vi "Dev List - Apply New.vi"(8 "error in (no error)":errorcluster, 9 "Dev Data Lookup Table in":variant, 10 "DataGridView in":refnum<class "DataGridView.lvclass">, 11 "Controller UI in":refnum<class "Controller UI.lvclass">) -> (0 "error out":errorcluster, 1 "Dev Data Lookup Table in out":variant, 2 "DataGridView out":refnum<class "DataGridView.lvclass">)   [LabVIEW 2016, in "Controller UI.lvlib" / "Controller UI.lvclass"]
uses:
  <userlib>/Common Components/Controller UI/Controller UI.lvclass
  C:/Program Files (x86)/National Instruments/LabVIEW 2016/vi.lib/ActorFramework/Actor/Actor.lvclass
  <userlib>/LabVIEWdotNetDataGrid/source/DataGridView/DataGridView.lvclass
  <vilib>/ActorFramework/Actor/Actor.lvclass/Actor.ctl
  <vilib>/ActorFramework/Message Enqueuer/Message Enqueuer.lvclass/Message Enqueuer.ctl
  <userlib>/Common Components/Hardware/DevInfo/DevInfo.lvclass
  <userlib>/Common Components/Controller UI/Dev Variant Data.ctl
  <userlib>/Common Components/Hardware/DevInfo/DevInfo.lvclass/DevInfo.ctl
  <userlib>/Common Components/Controller/Messages/Update a Dev Requested by UI Msg/Update a Dev Requested by UI Msg.lvclass/Update a Dev Requested by UI Msg.ctl
  <userlib>/Common Components/Hardware/DevInfo/Read GUID.vi
  <vilib>/ActorFramework/Message Enqueuer/Enqueue.vi
  <userlib>/Common Components/Controller Messages/Remove All Devices Msg/Remove All Devices Msg.lvclass
  C:/Program Files (x86)/National Instruments/LabVIEW 2016/vi.lib/ActorFramework/Message/Message.lvclass
  <userlib>/Common Components/Controller/Messages/Update a Dev Requested by UI Msg/Update a Dev Requested by UI Msg.lvclass
  <vilib>/ActorFramework/Message Priority Queue/Priority Enqueue.vi
  <userlib>/LabVIEWdotNetDataGrid/source/DataGridView/Get DataArray (String).vi
  <vilib>/ActorFramework/Actor/Actor.lvclass
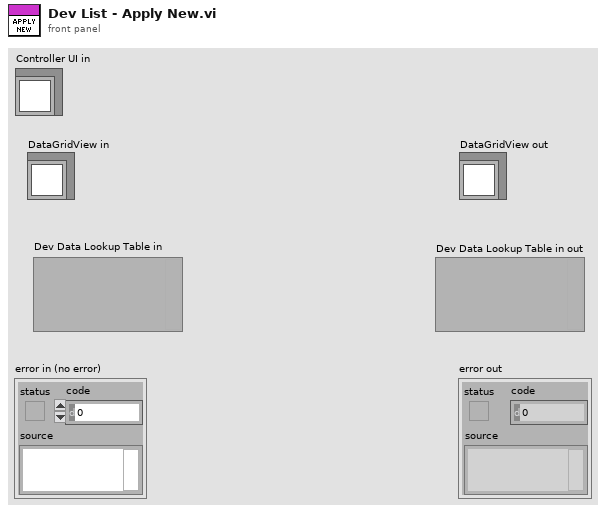
[diagram p1: front panel]
types:
  T1 = typedef "Controller UI.lvlib/Controller UI.lvclass/Dev Variant Data.ctl" = cluster{"Row Index":i32, "DevInfo Obj":refnum<class "DevInfo.lvclass">}
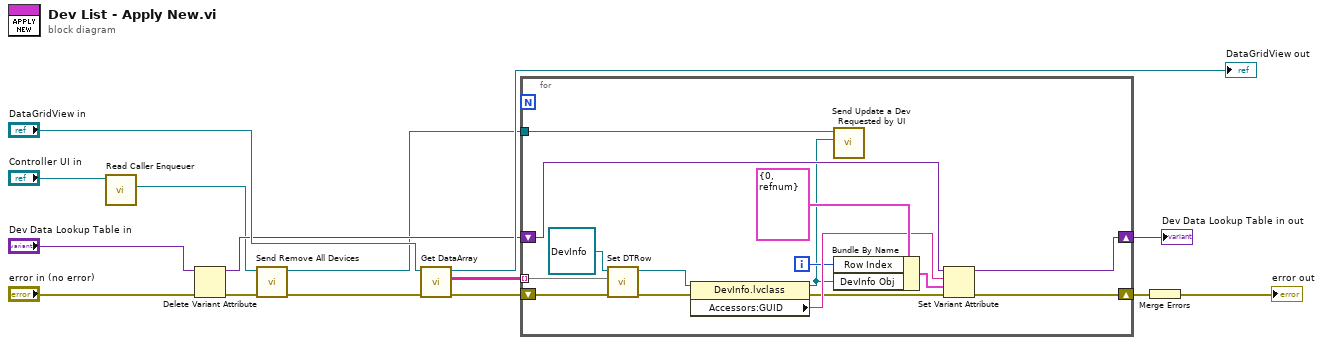
[diagram p0: block diagram]
diagram:
  n1 = call <vilib>:"Read Caller Enqueuer.vi"("Actor"="Controller UI in") -> ("Caller Enqueuer"=w2:refnum<class "Message Enqueuer.lvclass">)  [unwired: 10 in]
  n2 = Delete Variant Attribute(4:"error in (no error)", 7:"Dev Data Lookup Table in") -> (0:w6:errorcluster, 3:w9:variant)  [unwired: 1 in, 1 out]
  n3 = call <userlib>:"Send Remove All Devices.vi"("error in (no error)"=w6, "Message Enqueuer"=w2) -> ("error out"=w3:errorcluster, "Message Enqueuer out"=w1:refnum<class "Message Enqueuer.lvclass">)  [unwired: 8 in]
  n4 = call-poly <userlib>:"Get DataArray.vi"("error in (no error)"=w3, "DataGridView in"="DataGridView in") -> ("error out"=w5:errorcluster, "Array"=w14:string[][], "DataGridView out"=→"DataGridView out":refnum<class "DataGridView.lvclass">)  [unwired: 7 in]
  n5 = for {
    tunnel: w14 -> [w29] mode=indexing
    shift-right: [w19] -> w4
    shift-left: w5 -> [w27]
    shift-right: [w22] -> w8
    shift-left: w9 -> [w23]
    tunnel: w1 -> [w18]
    i -> [w17]
    n6 = call <userlib>:"Set DTRow.vi"("error in (no error)"=w27, "Dev Row Elements"=w29, "DevInfo in"=refnum<class "DevInfo.lvclass"> refnum ("DevInfo")) -> ("error out"=w26:errorcluster, "DevInfo out"=w28:refnum<class "DevInfo.lvclass">)  [unwired: 7 in]
    n7 = property class="DevInfo.lvclass"(reference=w28, error in=w26) -> (reference out=w16:refnum<class "DevInfo.lvclass">, error out=w20:errorcluster, "Accessors:GUID"=w21:string)
    n8 = call <userlib>:"Send Update a Dev Requested by UI.vi"("DevInfo"=w16, "Message Enqueuer in"=w18) -> ()  [unwired: 8 in, 2 out]
    n9 = Bundle By Name(cluster=T1 {"Row Index"=0, "DevInfo Obj"=refnum} ("Dev Data Lookup Table"), "Row Index"=w17, "DevInfo Obj"=w16) -> (w24:T1)
    n10 = Set Variant Attribute(Variant=w23, name=w21, value=w24, error in=w20) -> (Variant out=w22:variant, error out=w19:errorcluster)  [unwired: 1 out]
  }
  "Dev Data Lookup Table in out" <- w8
  n11 = Merge Errors(w4) -> (→"error out":errorcluster)
